vi "Set State.vi"(8 "error in (no error)":errorcluster, 10 "States":T1, 11 "Car Wash Controller Actor in":refnum<class "Car Wash Controller Actor.lvclass">) -> (0 "error out":errorcluster, 3 "Car Wash Controller Actor out":refnum<class "Car Wash Controller Actor.lvclass">)   [LabVIEW 2019, in "Car Wash Controller Actor.lvlib" / "Car Wash Controller Actor.lvclass"]
uses:
  Car Wash Controller Actor.lvclass
  State -Enum.ctl
  Car Wash Controller Actor.lvclass/Car Wash Controller Actor.ctl
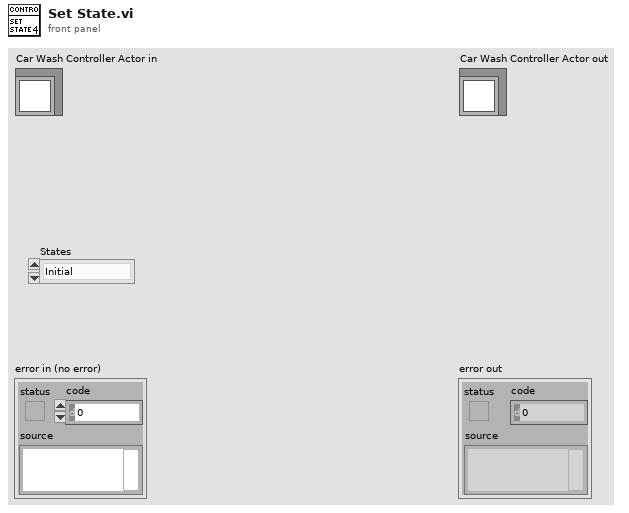
[diagram p1: front panel]
types:
  T1 = typedef "Car Wash Controller Actor.lvlib/Car Wash Controller Actor.lvclass/State -Enum.ctl" = enum16{"Initial", "Wait for Start", "Start", "Wait for Vehicle Position", "Wash Step Execution", "Wash Step/Cycle Completion", "Wash Exit", "Wash Abort/Terminate"}
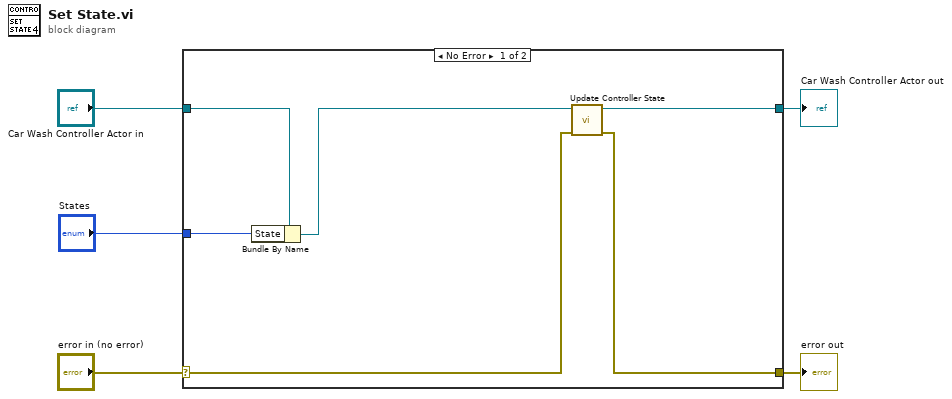
[diagram p0: block diagram]
diagram:
  n1 = case shown="No Error" "error in (no error)" {
    selector: "error in (no error)" -> [w7 w13]
    tunnel: [w6 w13] -> w4
    tunnel: [w8 w12] -> w2
    tunnel: "Car Wash Controller Actor in" -> [w11 w12]
    tunnel: "States" -> [w10 _]
    frame No Error {
      n2 = Bundle By Name(cluster=w11, "State"=w10) -> (w9:refnum<class "Car Wash Controller Actor.lvclass">)
      n3 = call "Update Controller State.vi"("error in (no error)"=w7, "Car Wash Controller Actor in"=w9) -> ("error out"=w6:errorcluster, "Car Wash Controller Actor out"=w8:refnum<class "Car Wash Controller Actor.lvclass">)  [unwired: 8 in]
    }
    frame Error {
    }
  }
  "error out" <- w4
  "Car Wash Controller Actor out" <- w2
